vi "Load.vi"(0 "Robot Event in":refnum<class "Robot Event.lvclass">, 1 "Event Parameters":T1[](array[typedef]), 5 "error in (no error)":errorcluster) -> (14 "Robot Event out":refnum<class "Robot Event.lvclass">, 19 "error out":errorcluster)   [LabVIEW 2019, in "Robot Event.lvclass"]
uses:
  Robot Event.lvclass
  Event Parameters.ctl
  Robot Event.lvclass/Robot Event.ctl
  <vilib>/regexp/Match Regular Expression.xnode
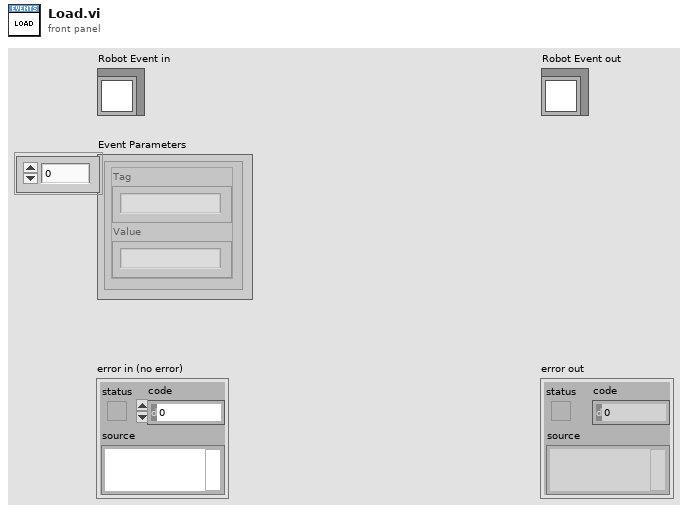
[diagram p1: front panel]
types:
  T1 = typedef "Robot Event.lvclass/Event Parameters.ctl" = cluster{"Tag":string, "Value":string}
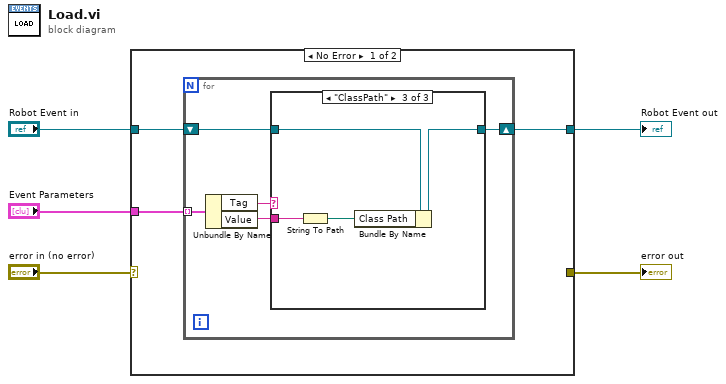
[diagram p0: block diagram]
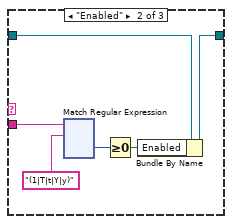
[diagram p3: hidden frame]
diagram:
  n1 = case shown="No Error" "error in (no error)" {
    selector: "error in (no error)" -> [_ w137]
    tunnel: [_ w137] -> w4
    tunnel: [w7 w136] -> w2
    tunnel: "Robot Event in" -> [w8 w136]
    tunnel: "Event Parameters" -> [w6 _]
    frame No Error {
      n2 = for {
        shift-right: [w12] -> w7
        shift-left: w8 -> [w13]
        tunnel: w6 -> [w11] mode=indexing
        n3 = Unbundle By Name(w11) -> ("Tag"=w10:string, "Value"=w9:string)
        n4 = case shown="\"ClassPath\"" w10 {
          tunnel: w13 -> [w14 w20 w135]
          tunnel: [w14 w19 w134] -> w12
          tunnel: w9 -> [_ w16 w133]
          frame Default {
          }
          frame "Enabled" {
            n5 = xnode "Match Regular Expression"("input string"=w16, "regular expression"="(1|T|t|Y|y)") -> ("offset past match"=w17:i32)  [unwired: 4 in, 4 out]
            n6 = Greater Or Equal To 0?(x=w17) -> (x >= 0?=w15:bool)
            n7 = Bundle By Name(cluster=w20, "Enabled"=w15) -> (w19:refnum<class "Robot Event.lvclass">)
          }
          frame "ClassPath" {
            n8 = String To Path(string=w133) -> (path=w132:path)
            n9 = Bundle By Name(cluster=w135, "Class Path"=w132) -> (w134:refnum<class "Robot Event.lvclass">)
          }
        }
      }
    }
    frame Error {
    }
  }
  "error out" <- w4
  "Robot Event out" <- w2
